vi "Convert String to Time Stamp.vi"(7 "default value of time stamp":timestamp, 11 "string":string) -> (3 "time stamp out":timestamp)   [LabVIEW 2013, in "infolib.lvlib"]
doc: "converts string to time stamp according ISO"
uses:
  infolib.lvlib
  <vilib>/Utility/miscctls.llb/LVDateTimeRec.ctl
  <vilib>/regexp/Match Regular Expression.xnode
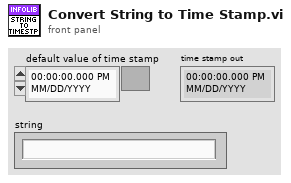
[diagram p1: front panel]
types:
  T1 = typedef "LVDateTimeRec.ctl" = cluster{"fractional second":dbl, "second":i32, "minute":i32, "hour":i32, "day of month":i32, "month":i32, "year":i32, "day of week":i32, "day of year":i32, "DST":i32}
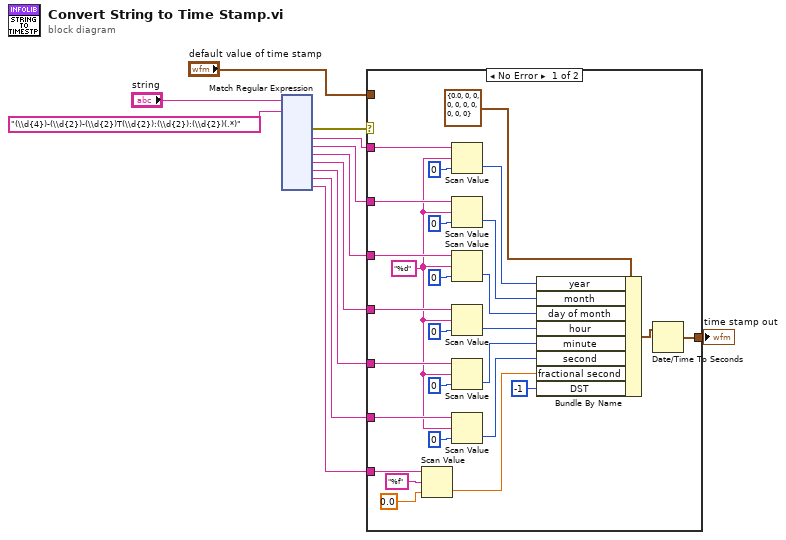
[diagram p0: block diagram]
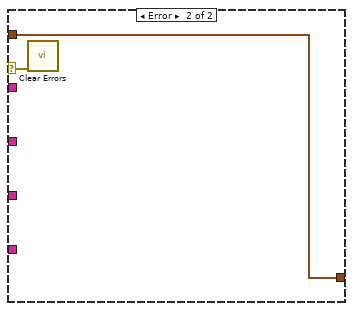
[diagram p2: hidden frame]
diagram:
  n1 = xnode "Match Regular Expression"("input string"="string", "regular expression"="(\\d{4})-(\\d{2})-(\\d{2})T(\\d{2}):(\\d{2}):(\\d{2})(.*)") -> ("error out"=w11:errorcluster, "submatch 1"=w3:string, "submatch 2"=w5:string, "submatch 3"=w6:string, "submatch 4"=w7:string, "submatch 5"=w8:string, "submatch 6"=w9:string, "submatch 7"=w10:string)  [unwired: 4 in, 4 out]
  n2 = case shown="No Error" w11 {
    selector: w11 -> [_ w41]
    tunnel: w3 -> [w39 _]
    tunnel: [w35 w40] -> w4
    tunnel: w5 -> [w31 _]
    tunnel: w6 -> [w29 _]
    tunnel: w7 -> [w26 _]
    tunnel: w8 -> [w23 _]
    tunnel: w9 -> [w20 _]
    tunnel: w10 -> [w17 _]
    tunnel: "default value of time stamp" -> [_ w40]
    frame No Error {
      w15 = "%d" ("format string")
      n3 = Scan Value(string=w17, format string="%f", default (0 dbl)=0.0) -> (value=w16:dbl)  [unwired: 1 out]
      n4 = Scan Value(string=w39, format string=w15, default (0 dbl)=0) -> (value=w33:i32)  [unwired: 1 out]
      n5 = Scan Value(string=w31, format string=w15, default (0 dbl)=0) -> (value=w32:i32)  [unwired: 1 out]
      n6 = Scan Value(string=w29, format string=w15, default (0 dbl)=0) -> (value=w28:i32)  [unwired: 1 out]
      n7 = Scan Value(string=w26, format string=w15, default (0 dbl)=0) -> (value=w25:i32)  [unwired: 1 out]
      n8 = Scan Value(string=w23, format string=w15, default (0 dbl)=0) -> (value=w22:i32)  [unwired: 1 out]
      n9 = Scan Value(string=w20, format string=w15, default (0 dbl)=0) -> (value=w19:i32)  [unwired: 1 out]
      n10 = Bundle By Name(cluster=T1 {"fractional second"=0.0, "second"=0, "minute"=0, "hour"=0, "day of month"=0, "month"=0, "year"=0, "day of week"=0, "day of year"=0, "DST"=0} ("date time rec"), "year"=w33, "month"=w32, "day of month"=w28, "hour"=w25, "minute"=w22, "second"=w19, "fractional second"=w16, "DST"=-1) -> (w34:T1)
      n11 = Date/Time To Seconds(2:w34) -> (0:w35:timestamp)  [unwired: 1 in]
    }
    frame Error {
      n12 = call <vilib>:"Clear Errors.vi"("error in (no error)"=w41) -> ()  [unwired: 6 in, 1 out]
    }
  }
  "time stamp out" <- w4
